vi "Get_Interrupt_Status.vi"(7 "I2C Channel":u8, 8 "error in":errorcluster, 10 "Interrupt Source":T1(ring), 11 "LINX Resource In":T3) -> (0 "error out":errorcluster, 2 "Interrupt Status":T2, 3 "LINX Resource Out":T3)   [LabVIEW 2014, in "LMH-LINX.lvlib" / "LIS331HH.lvlib"]
doc: "This VI provides information about where the interrupt(s) occured. Reading this register clears INT<1,2>_SRC IA bit (and the interrupt signal on INT<1,2> pin). Allows the refreshment of data in the INT<1,2>_SRC register if the lathed option was configured\n\n**Author: Stas Legedza"
uses:
  <vilib>/MakerHub/LINX/Public/Sensors/Accelerometer/LIS331HH/LIS331HH.lvlib
  <vilib>/MakerHub/LINX/Private/Type Defs/LINX Ref.ctl
  <vilib>/MakerHub/LINX/Private/Type Defs/Platform.ctl
  <vilib>/MakerHub/LINX/Private/Type Defs/Interface.ctl
  <vilib>/MakerHub/LINX/Private/Device/Type Defs/LINX Device Config.ctl
  <vilib>/MakerHub/LINX/Private/Device/Type Defs/TCP Config.ctl
  <vilib>/MakerHub/LINX/Private/Device/Type Defs/Channels.ctl
  <vilib>/MakerHub/LINX/Public/Sensors/Accelerometer/LIS331HH/_typeDefs/Interrupt_Status.ctl
  <vilib>/MakerHub/LINX/LMH-LINX.lvlib
  <vilib>/MakerHub/LINX/Private/Device/Device.lvlib
panel:
  # "INPUTS"
  # "OUTPUTS"
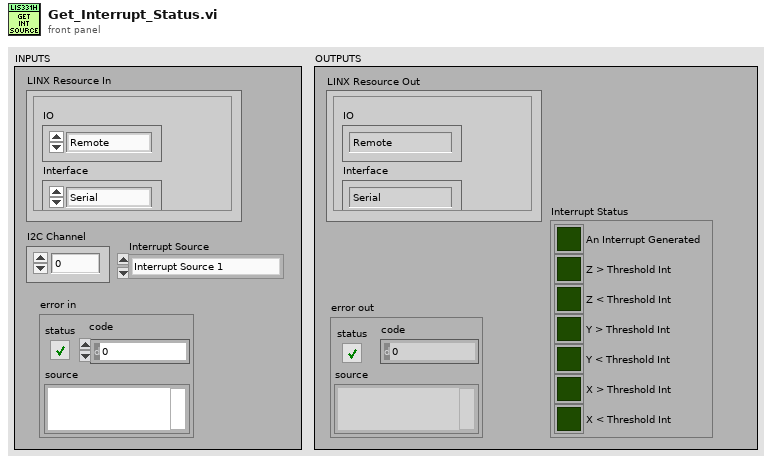
[diagram p1: front panel]
types:
  T1 = enum16{"Interrupt Source 1", "Interrupt Source 2"}
  T2 = typedef "LMH-LINX.lvlib/LIS331HH.lvlib/Interrupt_Status.ctl" = cluster{"An Interrupt Generated":bool, "Z > Threshold Int":bool, "Z < Threshold Int":bool, "Y > Threshold Int":bool, "Y < Threshold Int":bool, "X > Threshold Int":bool, "X < Threshold Int":bool}
  T3 = typedef "LMH-LINX.lvlib/LINX Ref.ctl" = cluster{"IO":T4, "Interface":T5, "LINX Device Config":T6}
  T4 = typedef "LMH-LINX.lvlib/Platform.ctl" = enum16{"Remote", "Local"}
  T5 = typedef "LMH-LINX.lvlib/Interface.ctl" = enum16{"Serial", "TCP"}
  T6 = typedef "LMH-LINX.lvlib/Device.lvlib/LINX Device Config.ctl" = cluster{"Interface":T5, "COM Port":refnum<visa-resource-name>, "TCP Configuration":T7, "Device Family":u8, "Device ID":u8, "Device Name":string, "TCP Ref":refnum<k5>, "Channels":T8}
  T7 = typedef "LMH-LINX.lvlib/Device.lvlib/TCP Config.ctl" = cluster{"IP Address":string, "Port":u16}
  T8 = typedef "LMH-LINX.lvlib/Channels.ctl" = cluster{"DI":u8[], "DO":u8[], "AI":u8[], "AO":u8[], "PWM":u8[], "QE":u8[], "UART":u8[], "I2C 2":u8[], "SPI":u8[], "CAN":u8[], "Servo":u8[], "AI Ref (V)":dbl, "AI Resolution (Bits)":u8, "AO Ref (V)":dbl, "AO Resolution (Bits)":u8}
  T9 = cluster{"Boolean array[0]":bool, "Boolean array[1]":bool, "Boolean array[2]":bool, "Boolean array[3]":bool, "Boolean array[4]":bool, "Boolean array[5]":bool, "Boolean array[6]":bool, "Boolean array[7]":bool}
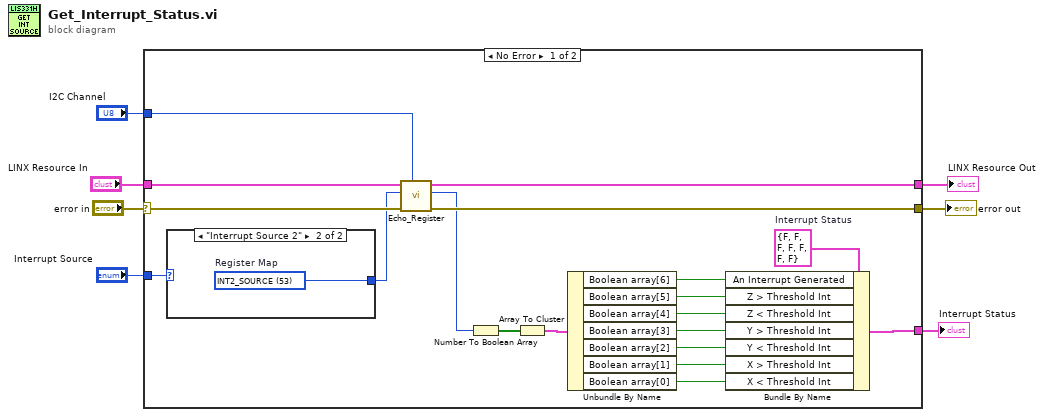
[diagram p0: block diagram]
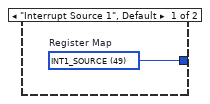
[diagram p2: hidden frame]
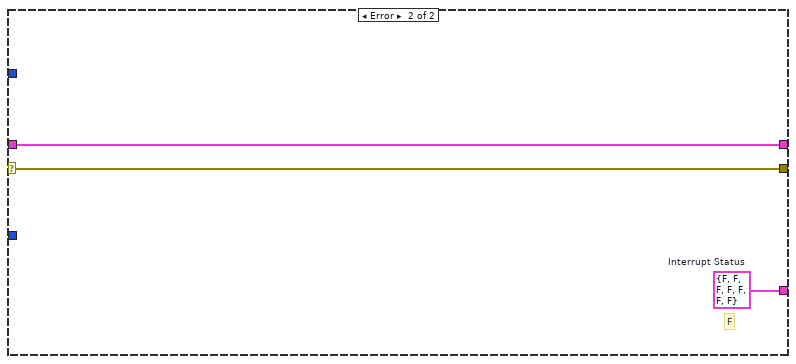
[diagram p3: hidden frame]
diagram:
  n1 = case shown="No Error" "error in" {
    selector: "error in" -> [w25 w31]
    tunnel: [w21 w31] -> w6
    tunnel: "LINX Resource In" -> [w26 w30]
    tunnel: "I2C Channel" -> [w24 _]
    tunnel: [w22 w30] -> w3
    tunnel: [w9 w29] -> w2
    tunnel: "Interrupt Source" -> [w8 _]
    frame No Error {
      w17 = T2 {"An Interrupt Generated"=FALSE, "Z > Threshold Int"=FALSE, "Z < Threshold Int"=FALSE, "Y > Threshold Int"=FALSE, "Y < Threshold Int"=FALSE, "X > Threshold Int"=FALSE, "X < Threshold Int"=FALSE}  # Interrupt Status
      n2 = case shown="\"Interrupt Source 2\"" w8 {
        tunnel: [w27 w28] -> w23
        frame "Interrupt Source 1", Default {
          w27 = u8 49 items=["CTRL_REG1"=32, "CTRL_REG2"=33, "CTRL_REG3"=34, "CTRL_REG4"=35, "CTRL_REG5"=36, "HP_FILTER_RESET"=37, "REFERENCE"=38, "STATUS_REG"=39, "OUT_X_L"=40, "OUT_X_H"=41, "OUT_Y_L"=42, "OUT_Y_H"=43, "OUT_Z_L"=44, "OUT_Z_H"=45, "INT1_CFG"=48, "INT1_SOURCE"=49, "INT1_THS"=50, "INT1_DURATION"=51, "INT2_CFG"=52, "INT2_SOURCE"=53, "INT2_THS"=54, "INT2_DURATION"=55]  # Register Map
        }
        frame "Interrupt Source 2" {
          w28 = u8 53 items=["CTRL_REG1"=32, "CTRL_REG2"=33, "CTRL_REG3"=34, "CTRL_REG4"=35, "CTRL_REG5"=36, "HP_FILTER_RESET"=37, "REFERENCE"=38, "STATUS_REG"=39, "OUT_X_L"=40, "OUT_X_H"=41, "OUT_Y_L"=42, "OUT_Y_H"=43, "OUT_Z_L"=44, "OUT_Z_H"=45, "INT1_CFG"=48, "INT1_SOURCE"=49, "INT1_THS"=50, "INT1_DURATION"=51, "INT2_CFG"=52, "INT2_SOURCE"=53, "INT2_THS"=54, "INT2_DURATION"=55]  # Register Map
        }
      }
      n3 = call <vilib>:"Echo_Register.vi"("I2C Channel"=w24, "error in (no error)"=w25, "Register to Echo"=w23, "LINX Resource In"=w26) -> ("error out"=w21:errorcluster, "Register Word"=w19:u8, "LINX Resource Out"=w22:T3)  [unwired: 5 in]
      n4 = Number To Boolean Array(number=w19) -> (Boolean array=w20:bool[])
      n5 = Array To Cluster(array=w20) -> (cluster=w18:T9)
      n6 = Unbundle By Name(w18) -> ("Boolean array[6]"=w16:bool, "Boolean array[5]"=w15:bool, "Boolean array[4]"=w14:bool, "Boolean array[3]"=w13:bool, "Boolean array[2]"=w12:bool, "Boolean array[1]"=w11:bool, "Boolean array[0]"=w10:bool)
      n7 = Bundle By Name(cluster=w17, "An Interrupt Generated"=w16, "Z > Threshold Int"=w15, "Z < Threshold Int"=w14, "Y > Threshold Int"=w13, "Y < Threshold Int"=w12, "X > Threshold Int"=w11, "X < Threshold Int"=w10) -> (w9:T2)
    }
    frame Error {
      w29 = T2 {"An Interrupt Generated"=FALSE, "Z > Threshold Int"=FALSE, "Z < Threshold Int"=FALSE, "Y > Threshold Int"=FALSE, "Y < Threshold Int"=FALSE, "X > Threshold Int"=FALSE, "X < Threshold Int"=FALSE}  # Interrupt Status
      # "F"
    }
  }
  "error out" <- w6
  "LINX Resource Out" <- w3
  "Interrupt Status" <- w2
